vi "PID Resize 1D Boolean Array.vi"(4 "array size":i32, 5 "input array":bool[](array[boolean])) -> (2 "output array":bool[](array[boolean]))   [LabVIEW 2017, in "NI_PID_pid.lvlib"]
uses:
  <vilib>/addons/control/pid/NI_PID_pid.lvlib
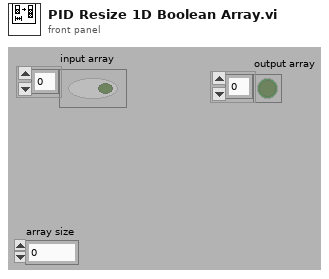
[diagram p1: front panel]
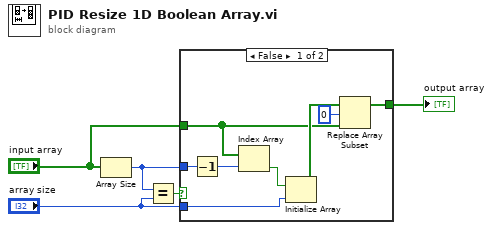
[diagram p0: block diagram]
diagram:
  n1 = Array Size(array="input array") -> (size(s)=w4:i32)
  n2 = Equal?(x=w4, y="array size") -> (x = y?=w5:bool)
  n3 = case shown="False" w5 {
    tunnel: "input array" -> [w7 w14]
    tunnel: [w12 w14] -> w1
    tunnel: "array size" -> [w10 _]
    tunnel: w4 -> [w13 _]
    frame False {
      n4 = Decrement(x=w13) -> (x-1=w11:i32)
      n5 = Index Array(array=w7, index=w11) -> (element=w9:bool)
      n6 = Initialize Array(w9, w10) -> (w8:bool[])
      n7 = Replace Array Subset(array=w8, new element=w7, index=0) -> (w12:bool[])
    }
    frame True {
    }
  }
  "output array" <- w1
